vi "SetSound.vi"(8 "error in (no error)":errorcluster, 11 "SnakeGame in":refnum<class "SnakeGame.lvclass">) -> (0 "error out":errorcluster, 3 "SnakeGame out":refnum<class "SnakeGame.lvclass">)   [LabVIEW 2019, in "RT_Game.lvlib" / "SnakeGame.lvclass"]
uses:
  SnakeGame.lvclass
  C:/Users/FreshBob/Dropbox/VIs/myRIO_GameConsole/RT/RT_Game/Game/Game.lvclass
  Menu/States.ctl
  Game/Game.lvclass/Game.ctl
  SnakeGame.lvclass/SnakeGame.ctl
  Snake/Snake.lvclass/Snake.ctl
  Game/Read State.vi
  Snake/Read Length.vi
  Snake/Read speed_multiplier.vi
  Snake/Read Dead_.vi
  Snake/Snake.lvclass
  Engine/Engine.lvclass
  Game/Game.lvclass
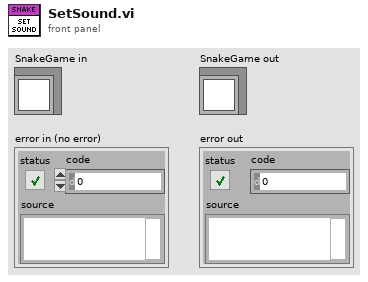
[diagram p1: front panel]
types:
  T1 = typedef "RT_Game.lvlib/Game.lvclass/States.ctl" = enum16{"Init", "Restart", "Menu", "Game", "Resume", "ToggleSingleplayer", "LoadNextGame", "ExitToMenu", "NewHighscore", "GameOver", "SlideOut", "FadeToMenu", "StartFadeToMenu"}
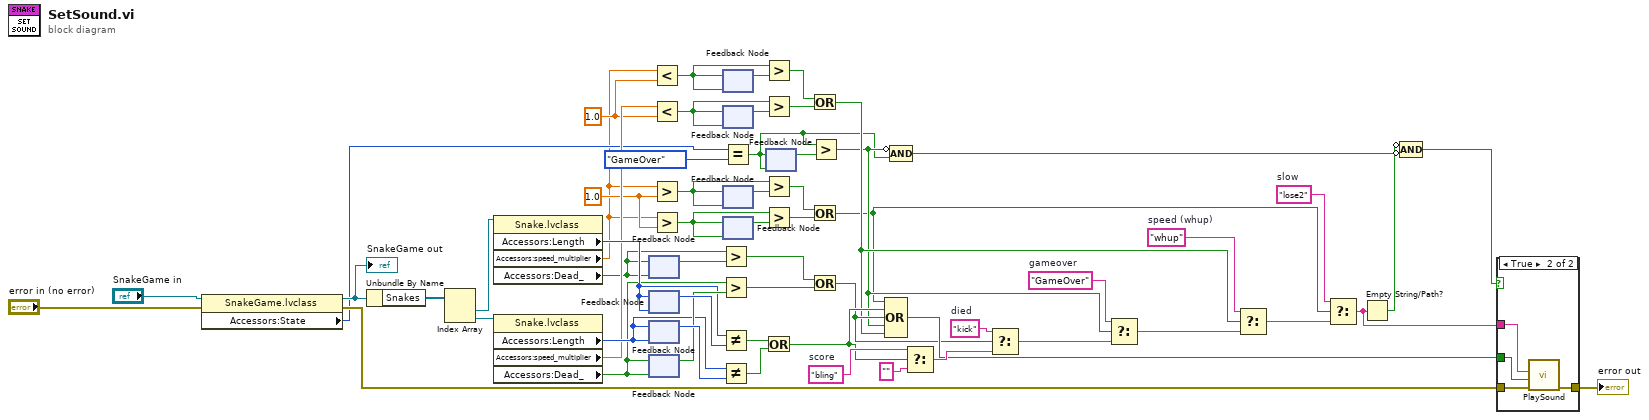
[diagram p0: block diagram]
diagram:
  w2 = "lose2"  # slow
  w12 = 1.0 ("x")
  w28 = 1.0 ("x")
  w43 = "whup"  # speed (whup)
  w47 = "GameOver"  # gameover
  w50 = "kick"  # died
  w52 = "bling"  # score
  n1 = property class="SnakeGame.lvclass"(reference="SnakeGame in", error in="error in (no error)") -> (reference out=w17:refnum<class "SnakeGame.lvclass">, error out=w19:errorcluster, "Accessors:State"=w16:T1)
  "SnakeGame out" <- w17
  n2 = Unbundle By Name(w17) -> ("Snakes"=w40:refnum<class "Snake.lvclass">[])
  n3 = Index Array(array=w40) -> (element #1=w39:refnum<class "Snake.lvclass">, element #2=w37:refnum<class "Snake.lvclass">)  [unwired: 2 in]
  n4 = property class="Snake.lvclass"(reference=w39) -> ("Accessors:Length"=w38:i16, "Accessors:speed_multiplier"=w11:dbl, "Accessors:Dead_"=w30:bool)  [unwired: 1 in, 2 out]
  n5 = property class="Snake.lvclass"(reference=w37) -> ("Accessors:Length"=w36:i16, "Accessors:speed_multiplier"=w33:dbl, "Accessors:Dead_"=w29:bool)  [unwired: 1 in, 2 out]
  n6 = feedback #1(w30) -> (w54:bool)
  n7 = feedback-in #1(w30) -> ()
  n8 = feedback-in #2(w38) -> ()
  n9 = feedback #2(w38) -> (w58:i16)
  n10 = feedback #3(w36) -> (w57:i16)
  n11 = feedback-in #3(w36) -> ()
  n12 = feedback #4(w29) -> (w53:bool)
  n13 = feedback-in #4(w29) -> ()
  n14 = Less?(x=w11, y=w28) -> (x < y?=w41:bool)
  n15 = Less?(x=w33, y=w28) -> (x < y?=w35:bool)
  n16 = Greater?(x=w11, y=w12) -> (0:w5:bool)
  n17 = Greater?(x=w11, y=w12) -> (0:w6:bool)
  n18 = Greater?(x=w30, y=w54) -> (0:w49:bool)
  n19 = Greater?(x=w29, y=w53) -> (0:w48:bool)
  n20 = Not Equal?(x=w38, y=w58) -> (x != y?=w56:bool)
  n21 = Not Equal?(x=w36, y=w57) -> (x != y?=w55:bool)
  n22 = feedback #5(w41) -> (w42:bool)
  n23 = feedback-in #5(w41) -> ()
  n24 = feedback #6(w35) -> (w34:bool)
  n25 = feedback-in #6(w35) -> ()
  n26 = Equal?(x=w16, y=States."GameOver") -> (x = y?=w15:bool)
  n27 = feedback #7(w5) -> (w7:bool)
  n28 = feedback-in #7(w5) -> ()
  n29 = feedback #8(w6) -> (w8:bool)
  n30 = feedback-in #8(w6) -> ()
  n31 = Greater?(x=w41, y=w42) -> (0:w31:bool)
  n32 = Greater?(x=w35, y=w34) -> (0:w32:bool)
  n33 = Greater?(x=w5, y=w7) -> (0:w10:bool)
  n34 = Greater?(x=w6, y=w8) -> (0:w9:bool)
  n35 = Or(x=w56, y=w55) -> (x .or. y?=w26:bool)
  n36 = feedback #9(w15) -> (w46:bool)
  n37 = feedback-in #9(w15) -> ()
  n38 = Or(x=w31, y=w32) -> (x .or. y?=w24:bool)
  n39 = Or(x=w10, y=w9) -> (x .or. y?=w1:bool)
  n40 = Or(x=w49, y=w48) -> (x .or. y?=w25:bool)
  n41 = Greater?(x=w15, y=w46) -> (0:w22:bool)
  n42 = Compound Arithmetic op=OR(w1, w26, w25, w22, w24) -> (w27:bool)
  n43 = Compound Arithmetic op=AND(invert w22, w15) -> (w45:bool)
  n44 = Select(t=w52, s=w26, f="") -> (s? t:f=w51:string)
  n45 = Select(t=w50, s=w25, f=w51) -> (s? t:f=w13:string)
  n46 = Select(t=w47, s=w22, f=w13) -> (s? t:f=w44:string)
  n47 = Select(t=w43, s=w24, f=w44) -> (s? t:f=w4:string)
  n48 = Select(t=w2, s=w1, f=w4) -> (s? t:f=w3:string)
  n49 = Empty String/Path?(string/path=w3) -> (empty?=w20:bool)
  n50 = Compound Arithmetic op=AND(invert w20, invert w45) -> (w21:bool)
  n51 = case shown="True" w21 {
    tunnel: w19 -> [w61 w65]
    tunnel: w27 -> [_ w64]
    tunnel: w3 -> [_ w63]
    tunnel: [w61 w62] -> w60
    frame False {
    }
    frame True {
      n52 = call "PlaySound.vi"("error in (no error)"=w65, "Overwrite"=w64, "Name"=w63) -> ("error out"=w62:errorcluster)  [unwired: 8 in]
    }
  }
  "error out" <- w60
